vi "Ej 7 Histograma.vi"() -> ()   [LabVIEW 2020]
uses:
  <vilib>/Instr/_visa.llb/VISA Configure Serial Port (Instr).vi
  <vilib>/ptbypt/NI_PtbyPt.lvlib
panel:
  in  "sample length":i32=100
  out "Cantidad de datos":i32
  out "Histogram Graph":T1(graph)
  in  "stop":bool
  out "Dato Leido":string
  in  "Seleccionar Puerto":refnum<visa-resource-name>
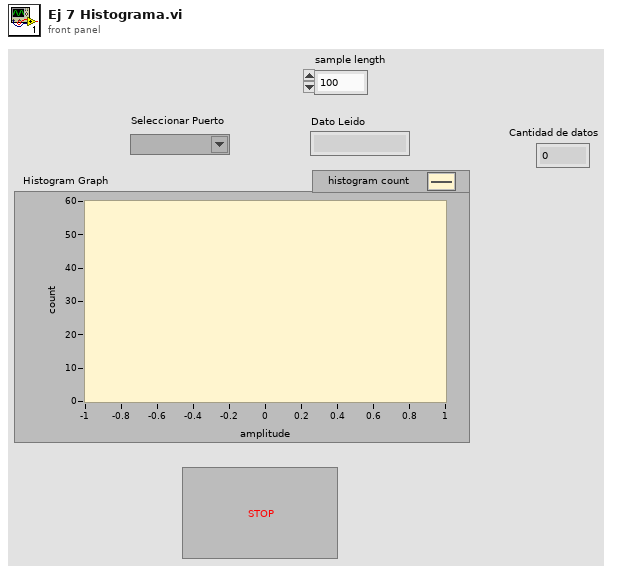
[diagram p1: front panel]
types:
  T1 = cluster{"X Values":dbl[], "Histogram: h(x)":i32[]}
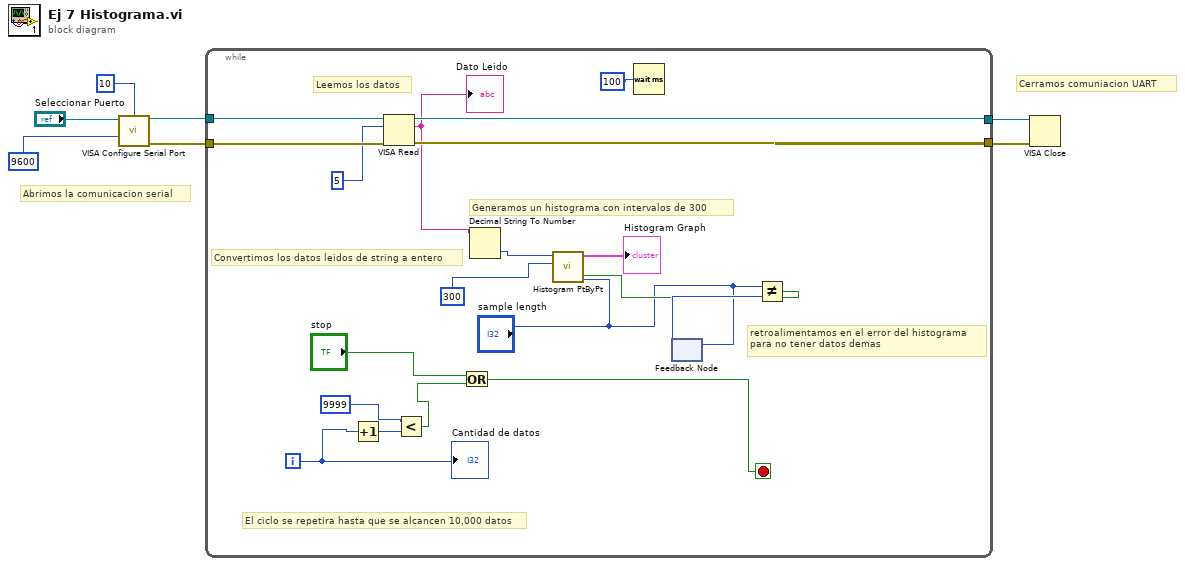
[diagram p0: block diagram]
diagram:
  # "Cerramos comuniacion UART"
  # "Abrimos la comunicacion serial"
  n1 = call-poly "VISA Configure Serial Port"("VISA resource name"="Seleccionar Puerto", "termination char\n(0xA = '\\n' = LF)"=u8 10 ("termination char\n(0xA = '\\n' = LF)"), "baud rate (9600)"=u32 9600) -> ("VISA resource name out"=w5:refnum<visa-resource-name>, "error out"=w4:errorcluster)  [unwired: 11 in]
  n2 = while {
    tunnel: w5 -> [w26]
    tunnel: w4 -> [w25]
    tunnel: [w22] -> w3
    tunnel: [w21] -> w2
    i -> [w9]
    stop <- w19 stop-if-true
    # "El ciclo se repetira hasta que se alcancen 10,000 datos"
    # "retroalimentamos en el error del histograma \npara no tener datos demas"
    # "Generamos un histograma con intervalos de 300"
    # "Convertimos los datos leidos de string a entero"
    # "Leemos los datos"
    n3 = Increment(x=w9) -> (x+1=w10:i32)
    n4 = VISA Read(VISA resource name=w26, byte count=u32 5, error in (no error)=w25) -> (VISA resource name out=w22:refnum<visa-resource-name>, read buffer=w14:string, error out=w21:errorcluster)  [unwired: 1 out]
    "Dato Leido" <- w14
    n5 = Less?(x=9999, y=w10) -> (x < y?=w11:bool)
    n6 = Or(x="stop", y=w11) -> (x .or. y?=w19:bool)
    n7 = Decimal String To Number(string=w14) -> (number=w13:i32)  [unwired: 2 in, 1 out]
    n8 = Wait (ms)(milliseconds to wait=u32 100) -> ()  [unwired: 1 out]
    n9 = feedback-in #1("sample length") -> ()
    n10 = feedback #1() -> (w16:i32)  [unwired: 1 in]
    n11 = Not Equal?(x="sample length", y=w16) -> (x != y?=w15:bool)
    n12 = call <vilib>:"Histogram PtByPt.vi"("initialize"=w15, "sample length"="sample length", "intervals"=300, "x"=w13) -> ("Histogram Graph"=→"Histogram Graph":T1)  [unwired: 4 in, 3 out]
    "Cantidad de datos" <- w9
  }
  n13 = VISA Close(VISA resource name=w3, error in (no error)=w2) -> ()  [unwired: 1 out]
